vi "GenerateTemporaryPath.vi"(8 "error in (no error)":errorcluster) -> (0 "error out":errorcluster, 3 "Unique Temporary File Path":path)   [LabVIEW 2010]
doc: "Returns a unique file path to the temporary directory. This VI only returns a path. It does not create the temporary file."
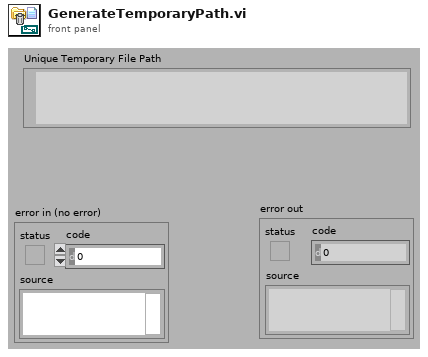
[diagram p1: front panel]
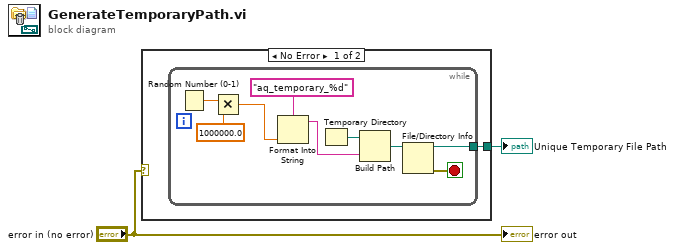
[diagram p0: block diagram]
diagram:
  n1 = case shown="No Error" "error in (no error)" {
    tunnel: [w3 _] -> w1
    frame No Error {
      n2 = while {
        tunnel: [w4] -> w3
        stop <- w5 stop-if-true
        n3 = Random Number (0-1)() -> (number: 0 to 1=w12:dbl)
        n4 = Multiply(x=w12, y=1000000.0) -> (x*y=w9:dbl)
        n5 = Format Into String(format string="aq_temporary_%d", w9) -> (resulting string=w8:string)  [unwired: 2 in, 1 out]
        n6 = Temporary Directory() -> (w7:path)
        n7 = Build Path(base path=w7, name or relative path=w8) -> (appended path=w6:path)
        n8 = File/Directory Info(path=w6) -> (path out=w4:path, error out=w5:errorcluster)  [unwired: 1 in, 5 out]
      }
    }
    frame Error {
    }
  }
  "Unique Temporary File Path" <- w1
  "error out" <- "error in (no error)"
